vi "Type Conversion.To Double.Subset (1D U8).vi"(9 "index (0)":i32, 10 "new values":u8[](array[numeric]), 11 "values in":dbl[](array[numeric])) -> (3 "values out":dbl[](array[numeric]))   [LabVIEW 2016, in "VeriStand Data.lvlib"]
doc: "Converts the provided values to double floats, preserving the numerical value of the data."
uses:
  VeriStand Data.lvlib
  Type Conversion.To Double (1D U8).vi
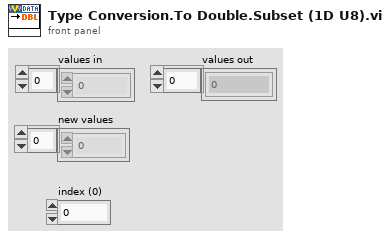
[diagram p1: front panel]
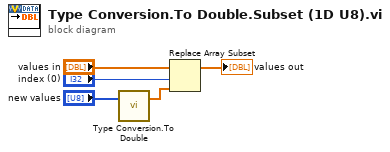
[diagram p0: block diagram]
diagram:
  n1 = call-poly "Type Conversion.To Double.vi"("values in"="new values") -> ("values out"=w1:dbl[])  [unwired: 2 in]
  n2 = Replace Array Subset(array="values in", new element=w1, index="index (0)") -> (→"values out":dbl[])
